vi "PH_ForceSensor.Calculate Status.vi"(0 "VI in":refnum<vi>, 5 "error in":errorcluster) -> (14 "VI out":refnum<vi>, 19 "error out":errorcluster)   [LabVIEW 2014, in "PH_ForceSensor.lvlib"]
uses:
  PH_ForceSensor.lvlib
  PH_Basics/PH_PP_Common/PH_PP_Common.PUs.ctl
  PH_Basics/PH_StatusHandler/PH_StatusHandler.Status.ctl
  PH_Basics/PH_StatusHandler/PH_StatusHandler.lvlib
  PHELIX/PH_BeamlineInformation/PH_BeamlineInformation.lvlib
  PH_Basics/PH_PP_Common/PH_PP_Common.lvlib
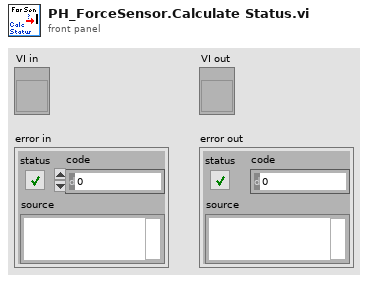
[diagram p1: front panel]
types:
  T1 = typedef "PH_StatusHandler.lvlib/PH_StatusHandler.Status.ctl" = i16
  T2 = typedef "PH_PP_Common.lvlib/PH_PP_Common.PUs.ctl" = enum16{"no Info", "PA-19mm-1", "PA-19mm-2", "PA-45mm-PILC", "PA-45mm-MAIN", "MA-PU-1", "MA-PU-2", "MA-PU-3", "MA-PU-4", "MA-PU-5", "MA-PU-6", "MA-FR", "MA-PILC", "PA-45mm-DP"}
  T3 = typedef "PH_ForceSensor.lvlib/PH_ForceSensor.i attribute.ctl" = cluster{"GUI Refs":T4, "Rawvalues":T5, "Offsets [µV]":T5, "Scalings [mV/V]":T5, "Forces [N]":T5, "Supply Voltage [V]":dbl, "Full Force [N]":dbl, "Ranges [N]":cluster{"Low Energy":cluster{"Upper Limit":dbl, "Lower Limit":dbl}, "High Energy":cluster{"Upper Limit":dbl, "Lower Limit":dbl}}}
  T4 = typedef "PH_ForceSensor.lvlib/PH_ForceSensor.GUI Refs.ctl" = cluster{"Delete":refnum<vi>, "Rawvalues":refnum<vi>, "Offsets [µV]":refnum<vi>, "Sensor Values [µV]":refnum<vi>, "Scalings [mV/V]":refnum<vi>, "Supply Voltage [V]":refnum<vi>, "Full Force [N]":refnum<vi>, "Forces [N]":refnum<vi>, "Graph Differential Forces":refnum<vi>, "Graph Absolute Forces":refnum<vi>, "Ranges [N]":refnum<vi>}
  T5 = typedef "PH_ForceSensor.lvlib/PH_ForceSensor.Dataset.ctl" = cluster{"top front":dbl, "top back":dbl, "bottom front":dbl, "bottom back":dbl}
  T6 = typedef "PH_BeamlineInformation.lvlib/PH_BeamlineInformation.i attribute.ctl" = cluster{"BL GUI Elements of Services":cluster{"Service Name":string, "GUI Elements":refnum<vi>[], "Status":i32}[], "Powermeters":T7, "Efficiency":T8, "Heads":T9[]}
  T7 = typedef "PH_BeamlineInformation.lvlib/PH_BeamlineInformation.Powermeter.ctl" = cluster{"ns FE":cluster{"GUI Ref":refnum<vi>, "Value":dbl}, "fs FE":cluster{"GUI Ref":refnum<vi>, "Value":dbl}, "PA":cluster{"GUI Ref":refnum<vi>, "Value":dbl}, "MA":cluster{"GUI Ref":refnum<vi>, "Value":dbl}, "Z6 green":cluster{"GUI Ref":refnum<vi>, "Value":dbl}, "Z6 IR":cluster{"GUI Ref":refnum<vi>, "Value":dbl}, "Z6 COS":cluster{"GUI Ref":refnum<vi>, "Value":dbl}}
  T8 = typedef "PH_BeamlineInformation.lvlib/PH_BeamlineInformation.Efficiency.ctl" = cluster{"PA Gain":cluster{"GUI Ref":refnum<vi>, "Value":dbl}, "MA Gain":cluster{"GUI Ref":refnum<vi>, "Value":dbl}, "Z6 green Conversion":cluster{"GUI Ref":refnum<vi>, "Value":dbl}, "Z6 Comp Losses":cluster{"GUI Ref":refnum<vi>, "Value":dbl}}
  T9 = typedef "PH_BeamlineInformation.lvlib/PH_BeamlineInformation.Head.ctl" = cluster{"PowerUnit":T2, "in use":cluster{"Value":bool, "GUI Ref":refnum<vi>, "linked":bool}, "voltage":cluster{"Value":dbl, "GUI Ref":refnum<vi>, "linked":bool}}
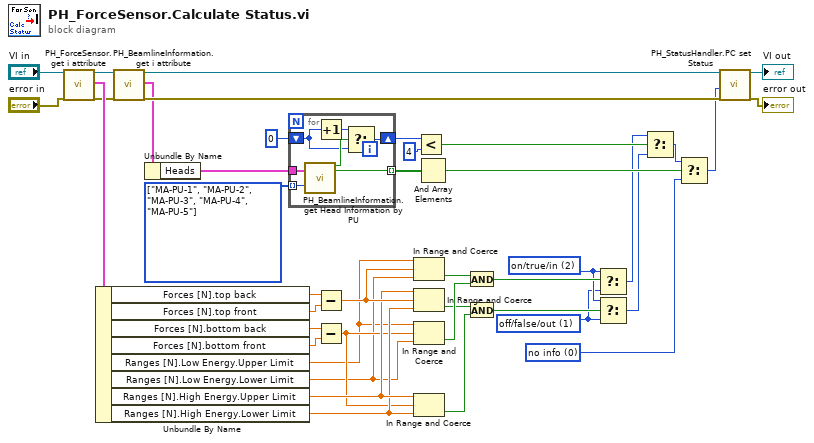
[diagram p0: block diagram]
diagram:
  w4 = T1 1 items=["no info", "off/false/out", "on/true/in", "Failure", "Alarm", "Status 1", "Status 2", "Status 3"] ("f")
  w5 = T1 2 items=["no info", "off/false/out", "on/true/in", "Failure", "Alarm", "Status 1", "Status 2", "Status 3"] ("Status")
  w12 = T1 0 items=["no info", "off/false/out", "on/true/in", "Failure", "Alarm", "Status 1", "Status 2", "Status 3"] ("Status")
  w30 = T2[] [enum."MA-PU-1", enum."MA-PU-2", enum."MA-PU-3", enum."MA-PU-4", enum."MA-PU-5"] items=["no Info", "PA-19mm-1", "PA-19mm-2", "PA-45mm-PILC", "PA-45mm-MAIN", "MA-PU-1", "MA-PU-2", "MA-PU-3", "MA-PU-4", "MA-PU-5", "MA-PU-6", "MA-FR", "MA-PILC", "PA-45mm-DP"]
  n1 = call "PH_ForceSensor.get i attribute.vi"("i ref in"="VI in", "error in (no error)"="error in") -> ("i ref out"=w36:refnum<vi>, "i attribute"=w39:T3, "error out"=w34:errorcluster)  [unwired: 15 in]
  n2 = Unbundle By Name(w39) -> ("Forces [N].top back"=w24:dbl, "Forces [N].top front"=w22:dbl, "Forces [N].bottom back"=w23:dbl, "Forces [N].bottom front"=w21:dbl, "Ranges [N].Low Energy.Upper Limit"=w1:dbl, "Ranges [N].Low Energy.Lower Limit"=w16:dbl, "Ranges [N].High Energy.Upper Limit"=w19:dbl, "Ranges [N].High Energy.Lower Limit"=w18:dbl)
  n3 = call "PH_BeamlineInformation.get i attribute.vi"("i ref in"=w36, "error in (no error)"=w34) -> ("i ref out"=w35:refnum<vi>, "i attribute"=w32:T6, "error out"=w33:errorcluster)  [unwired: 15 in]
  n4 = Unbundle By Name(w32) -> ("Heads"=w31:T9[])
  n5 = for {
    tunnel: w31 -> [w48]
    tunnel: w30 -> [w47] mode=indexing
    tunnel: [w46] -> w29 mode=indexing
    shift-right: [w43] -> w27
    shift-left: 0 -> [w42]
    n6 = call "PH_BeamlineInformation.get Head Information by PU.vi"("Heads"=w48, "Power Unit"=w47) -> ("In Use?"=w45:bool, "In Use linked?"=w46:bool)  [unwired: 12 in, 4 out]
    n7 = Increment(x=w42) -> (x+1=w44:i32)
    n8 = Select(t=w44, s=w45, f=w42) -> (s? t:f=w43:i32)
  }
  n9 = Subtract(x=w24, y=w22) -> (x-y=w20:dbl)
  n10 = Subtract(x=w23, y=w21) -> (x-y=w17:dbl)
  n11 = In Range and Coerce(upper limit=w1, x=w20, lower limit=w16) -> (In Range?=w15:bool)  [unwired: 1 out]
  n12 = In Range and Coerce(upper limit=w19, x=w20, lower limit=w18) -> (In Range?=w8:bool)  [unwired: 1 out]
  n13 = In Range and Coerce(upper limit=w1, x=w17, lower limit=w16) -> (In Range?=w14:bool)  [unwired: 1 out]
  n14 = In Range and Coerce(upper limit=w19, x=w17, lower limit=w18) -> (In Range?=w7:bool)  [unwired: 1 out]
  n15 = Less?(x=w27, y=4 ("x")) -> (x < y?=w25:bool)
  n16 = And Array Elements(Boolean array=w29) -> (logical AND=w13:bool)
  n17 = And(x=w15, y=w14) -> (x .and. y?=w10:bool)
  n18 = And(x=w8, y=w7) -> (x .and. y?=w6:bool)
  n19 = Select(t=w5, s=w10, f=w4) -> (s? t:f=w9:T1)
  n20 = Select(t=w5, s=w6, f=w4) -> (s? t:f=w3:T1)
  n21 = Select(t=w9, s=w25, f=w3) -> (s? t:f=w2:T1)
  n22 = Select(t=w2, s=w13, f=w12) -> (s? t:f=w11:T1)
  n23 = call "PH_StatusHandler.PC set Status.vi"("i ref in"=w35, "Status"=w11, "error in (no error)"=w33) -> ("i ref out"=→"VI out":refnum<vi>, "error out"=→"error out":errorcluster)  [unwired: 15 in]
